vi "SUB_Relay_RTN_Low.vi"(2 "element":T1(array[cluster])) -> ()   [LabVIEW 2011]
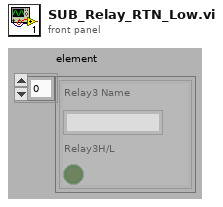
[diagram p1: front panel]
types:
  T1 = cluster{"Relay3 Name":string, "Relay3H/L":bool}[]
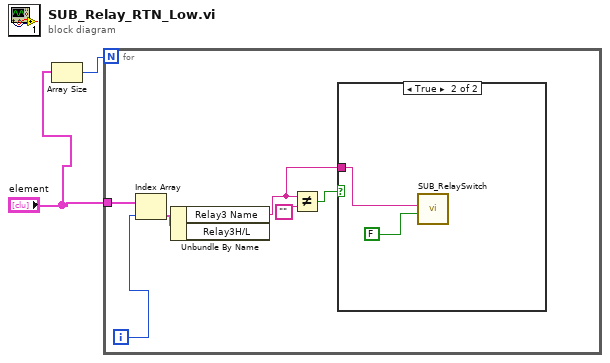
[diagram p0: block diagram]
diagram:
  n1 = Array Size(array="element") -> (size(s)=w1:i32)
  n2 = for {
    N: w1 -> [_]
    tunnel: "element" -> [w5]
    i -> [w7]
    n3 = Index Array(array=w5, index=w7) -> (element=w3:cluster{"Relay3 Name":string, "Relay3H/L":bool})
    n4 = Unbundle By Name(w3) -> ("Relay3 Name"=w4:string)  [unwired: 1 out]
    n5 = Not Equal?(x=w4, y="") -> (x != y?=w6:bool)
    n6 = case shown="True" w6 {
      tunnel: w4 -> [_ w10]
      frame False {
      }
      frame True {
        n7 = call "SUB_RelaySwitch.vi"("ON_OFF"=FALSE, "DIO"=w10) -> ()  [unwired: 2 in, 1 out]
      }
    }
  }
